vi "Destroy.vi"(8 "error in (no error)":errorcluster, 11 "gRPC service in":refnum<class "streamai.lvclass">) -> (0 "error out":errorcluster, 3 "gRPC service out":refnum<class "streamai.lvclass">)   [LabVIEW 2023, in "Generated_server.lvlib" / "streamai.lvclass"]
uses:
  streamai.lvclass
  streamai.lvclass/streamai.ctl
  <vilib>/gRPC/LabVIEW gRPC Servicer/ServiceBase/ServiceBase.lvclass
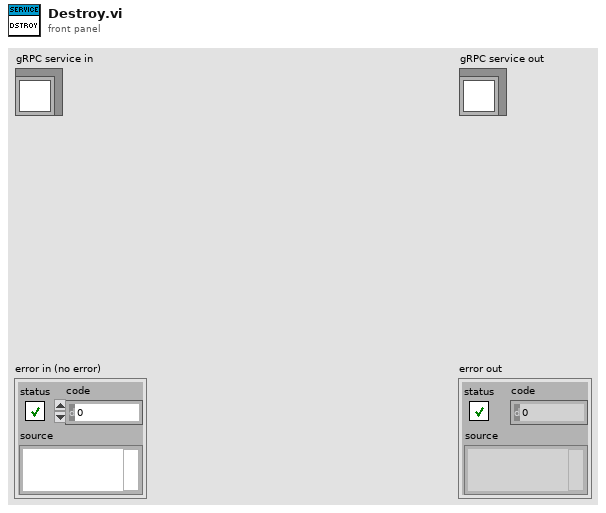
[diagram p1: front panel]
types:
  T1 = typedef "Generated_server.lvlib/streamai.lvclass/Server gRPC UEs.ctl" = cluster{"streamai startacq gRPC UE":refnum<user-event>, "streamai stopacq gRPC UE":refnum<user-event>, "streamai setSignalConfig gRPC UE":refnum<user-event>, "streamai setSamplingConfig gRPC UE":refnum<user-event>}
  T2 = typedef "Generated_server.lvlib/streamai.lvclass/Server Internal UEs.ctl" = cluster{"streamai startacq Internal UE":refnum<user-event>, "streamai stopacq Internal UE":refnum<user-event>, "streamai setSignalConfig Internal UE":refnum<user-event>, "streamai setSamplingConfig Internal UE":refnum<user-event>}
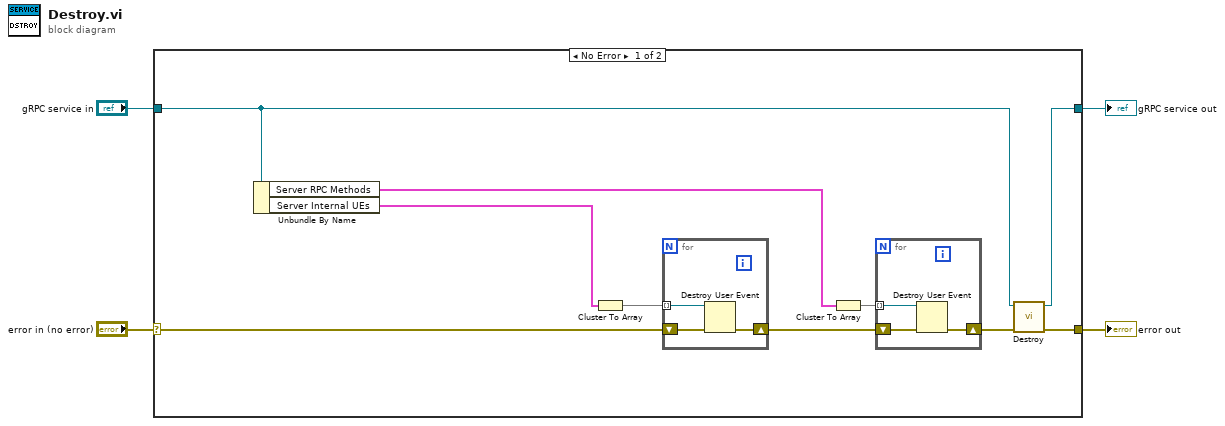
[diagram p0: block diagram]
diagram:
  n1 = case shown="No Error" "error in (no error)" {
    selector: "error in (no error)" -> [w9 w22]
    tunnel: [w5 w22] -> w3
    tunnel: [w7 w21] -> w1
    tunnel: "gRPC service in" -> [w8 w21]
    frame No Error {
      n2 = Unbundle By Name(w8) -> ("Server RPC Methods"=w12:T1, "Server Internal UEs"=w13:T2)
      n3 = Cluster To Array(cluster=w13) -> (array=w14:refnum<user-event>[])
      n4 = for {
        tunnel: w14 -> [w20] mode=indexing
        shift-right: [w18] -> w10
        shift-left: w9 -> [w19]
        n5 = Destroy User Event(user event=w20, error in=w19) -> (error out=w18:errorcluster)
      }
      n6 = Cluster To Array(cluster=w12) -> (array=w11:refnum<user-event>[])
      n7 = for {
        tunnel: w11 -> [w17] mode=indexing
        shift-right: [w15] -> w6
        shift-left: w10 -> [w16]
        n8 = Destroy User Event(user event=w17, error in=w16) -> (error out=w15:errorcluster)
      }
      n9 = call-parent "Destroy.vi"("error in"=w6, "gRPC service in"=w8) -> ("error out"=w5:errorcluster, "gRPC service out"=w7:refnum<class "streamai.lvclass">)  [unwired: 8 in]
    }
    frame Error {
    }
  }
  "error out" <- w3
  "gRPC service out" <- w1
